vi "SubVI Tester.vi"() -> ()   [LabVIEW 2015]
uses:
  Weather Data.ctl
panel:
  in  "Weather Data In":T1
  out "Weather Data Out":T1
  out "Thermometer":dbl(slide) scale=0.0..100.0
  in  "Min Temperature":dbl=10.0
  in  "Max Temperature":dbl=30.0
  in  "Stop":bool
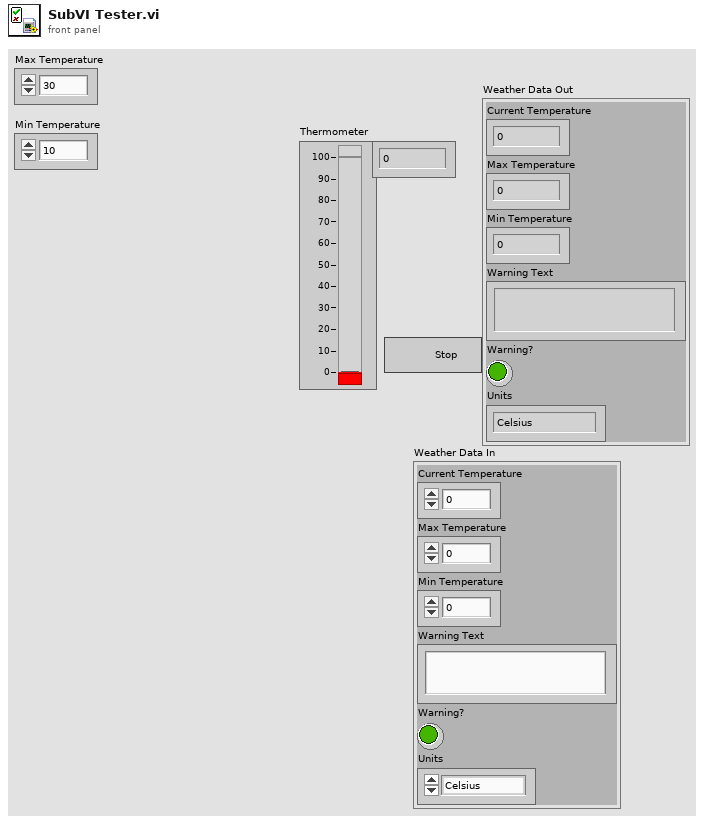
[diagram p1: front panel]
types:
  T1 = typedef "Weather Data.ctl" = cluster{"Current Temperature":dbl, "Max Temperature":dbl, "Min Temperature":dbl, "Warning Text":string, "Warning?":bool, "Units":enum16{"Celsius", "Faharenheit"}}
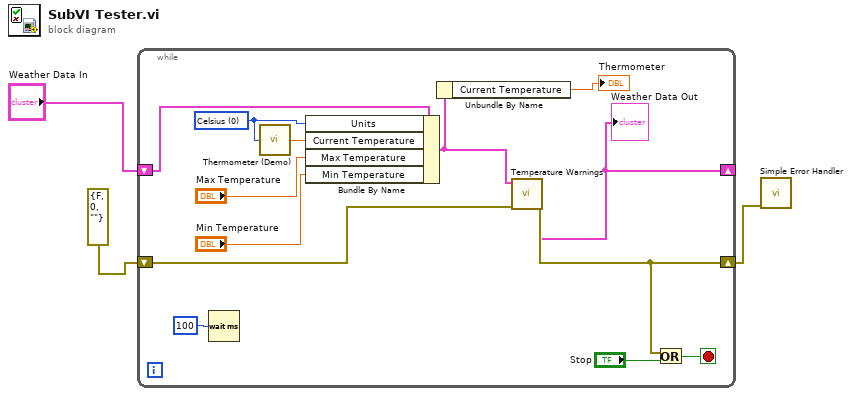
[diagram p0: block diagram]
diagram:
  n1 = while {
    shift-right: [w12] -> w3
    shift-left: errorcluster {"status"=FALSE, "code"=0, "source"=""} ("error out") -> [w13]
    shift-right: [w5] -> _
    shift-left: "Weather Data In" -> [w7]
    stop <- w14 stop-if-true
    w6 = u16 0 items=["Celsius", "Fahrenheit"] ("Units (0: Celsius)")
    n2 = Wait (ms)(milliseconds to wait=u32 100) -> ()  [unwired: 1 out]
    n3 = call "Thermometer (Demo).vi"("Units (0: Celsius)"=w6) -> ("Temperature Value"=w11:dbl)
    n4 = Bundle By Name(cluster=w7, "Units"=w6, "Current Temperature"=w11, "Max Temperature"="Max Temperature", "Min Temperature"="Min Temperature") -> (w4:T1)
    n5 = Unbundle By Name(w4) -> ("Current Temperature"=→"Thermometer":dbl)
    n6 = call "Temperature Warnings.vi"("Error In"=w13, "Weather Data In"=w4) -> ("Error Out"=w12:errorcluster, "Weather Data Out"=w5:T1)  [unwired: 8 in]
    "Weather Data Out" <- w5
    n7 = Or(x=w12, y="Stop") -> (x .or. y?=w14:bool)
  }
  n8 = call <vilib>:"Simple Error Handler.vi"("error in (no error)"=w3) -> ()  [unwired: 4 in, 5 out]
